vi "Test Event.vi"(8 "error in (no error)":errorcluster, 9 "Source":T1=enum."Unknown") -> (0 "error out":errorcluster, 3 "Events out":refnum<class "Event.lvclass">)   [LabVIEW 2019, in "Event.lvclass"]
uses:
  Event.lvclass
  C:/Projekty/_Wewnetrzne/PC_ActorFramework/07_Program/LABVIEW/02_Source/Classes/EventsAbstract/EventsAbstract.lvclass
  SubModules/LogsAbstract/TypeDef/Event Source.ctl
  TypeDef/Event Classification.ctl
  Event.lvclass/Event.ctl
  fd706440-9d0c-449a-a399-c2c596811bd4.vi
  SubModules/EventLog Messages/Enqueue Logs Element Msg/Send Enqueue Logs Element.vi
  <vilib>/ActorFramework/Message Enqueuer/Enqueue.vi
  <vilib>/Utility/Data Type/Get Numeric Information.vi
  EventsAbstract/sVI/Actual Date and Time.vi
  EventsAbstract/Accessors/Read Info.vi
  EventsAbstract/Accessors/Write Info.vi
  EventsAbstract/Accessors/Write Actions.vi
  SubModules/EventLog/FGV+Globals/EventLogRef Global.vi
  <vilib>/ActorFramework/Message Priority Queue/Priority Enqueue.vi
  <vilib>/ActorFramework/Message Enqueuer/Message Enqueuer.lvclass
  EventsAbstract/EventsAbstract.lvclass
  SubModules/EventLog Messages/Enqueue Logs Element Msg/Enqueue Logs Element Msg.lvclass
  SubModules/LogsAbstract/LogsAbstract.lvclass
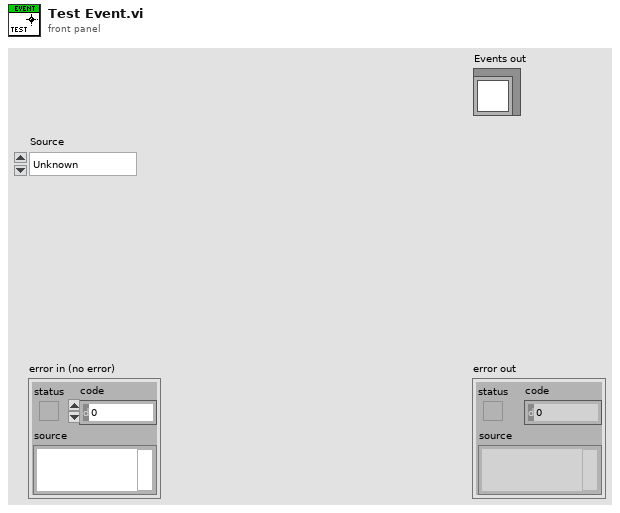
[diagram p1: front panel]
types:
  T1 = typedef "LogsAbstract.lvlib/LogsAbstract.lvclass/Event Source.ctl" = enum16{"LabView Call Chain", "Unknown", "< --- Modules --- >", "Core", "< --- SubModules --- >", "EventLog -> Core", "ErrorLog -> Core"}
  T2 = typedef "Event.lvclass/Event Classification.ctl" = enum16{"System Log", "test1", "test2", "test3"}
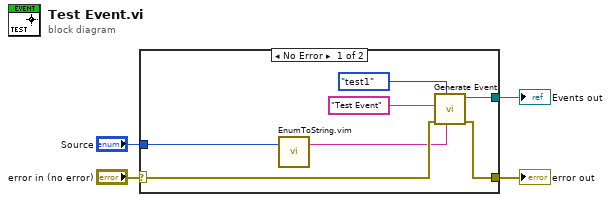
[diagram p0: block diagram]
diagram:
  n1 = case shown="No Error" "error in (no error)" {
    selector: "error in (no error)" -> [w9 w12]
    tunnel: [w8 w12] -> w3
    tunnel: [w11 _] -> w2
    tunnel: "Source" -> [w6 _]
    frame No Error {
      n2 = call "EnumToString.vim"("Enum"=w6) -> ("Enum Value"=w5:string)  [unwired: 16 in, 2 out]
      n3 = call "Generate Event.vi"("Source"=w5, "Classification"=Event_Classification."test1", "Error In"=w9, "Description"="Test Event") -> ("Error Out"=w8:errorcluster, "Events out"=w11:refnum<class "Event.lvclass">)  [unwired: 6 in]
    }
    frame Error {
    }
  }
  "error out" <- w3
  "Events out" <- w2
